vi "rsscope_core_global.vi"() -> ()   [LabVIEW 2018] (continued)
condition In Range or Out of Range.\n\nAvailable Repeated Capabilities:\nTrigger: TrigA, TrigB, TrigR\r\n\nRemote-control command(s):\nTRIGger<m>:DPHY:ESINdex:MAX"}, {"Level"=3, "Class Only"=TRUE, "Identifier"="", "Descriptive Name"="Escape Mode", "Data Type"=0, "Command"="", "Access"=0, "Range Table"="", "Read Callback"="", "Write Callback"="", "Supported Models"="", "Instrument Options"="", "Flags"=0, "Help"="Set the specified data value to be triggered on.The escape mode setup consists of the condition and one or two data patterns."}, {"Level"=4, "Class Only"=FALSE, "Identifier"="RSSCOPE_ATTR_DPHY_TRIGGER_ESCAPE_MODE_CONDITION", "Descriptive Name"="DPHY Trigger Escape Mode Condition", "Data Type"=0, "Command"="TRIG{Trigger}:DPHY:ESCM:COND", "Access"=2, "Range Table"="rsscope_rngProtocolTriggerCondition", "Read Callback"="", "Write Callback"="", "Supported Models"="", "Instrument Options"="K42", "Flags"=0, "Help"="Set the condition for the escape mode. You can define an exact value or a value range.\n\nAvailable Repeated Capabilities:\nTrigger: TrigA, TrigB, TrigR\r\n\nRemote-control command(s):\nTRIGger<m>:DPHY:ESCMode:CONDition"}, {"Level"=4, "Class Only"=FALSE, "Identifier"="RSSCOPE_ATTR_DPHY_TRIGGER_ESCAPE_MODE_MIN", "Descriptive Name"="DPHY Trigger Escape Mode Min", "Data Type"=2, "Command"="TRIG{Trigger}:DPHY:ESCM:MIN", "Access"=2, "Range Table"="", "Read Callback"="", "Write Callback"="", "Supported Models"="", "Instrument Options"="K42", "Flags"=0, "Help"="Specifies a escape mode bit pattern, or sets the start value of a pattern range.\n\nValid Values:\nBinary pattern string consisting of 1; 0; or X (any bit).\n\nAvailable Repeated Capabilities:\nTrigger: TrigA, TrigB, TrigR\r\n\nRemote-control command(s):\nTRIGger<m>:DPHY:ESCMode:MIN"}, {"Level"=4, "Class Only"=FALSE, "Identifier"="RSSCOPE_ATTR_DPHY_TRIGGER_ESCAPE_MODE_MAX", "Descriptive Name"="DPHY Trigger Escape Mode Max", "Data Type"=2, "Command"="TRIG{Trigger}:DPHY:ESCM:MAX", "Access"=2, "Range Table"="", "Read Callback"="", "Write Callback"="", "Supported Models"="", "Instrument Options"="K42", "Flags"=0, "Help"="Sets the end value of an escape mode range for condition In Range or Out of Range. \n\nValid Values:\nBinary pattern string consisting of 1; 0; or X (any bit).\n\nAvailable Repeated Capabilities:\nTrigger: TrigA, TrigB, TrigR\r\n\nRemote-control command(s):\nTRIGger<m>:DPHY:ESCMode:MAX"}, {"Level"=2, "Class Only"=TRUE, "Identifier"="", "Descriptive Name"="M-PHY", "Data Type"=0, "Command"="", "Access"=0, "Range Table"="", "Read Callback"="", "Write Callback"="", "Supported Models"="", "Instrument Options"="", "Flags"=0, "Help"="Contains attributes for M-PHY triggering."}, {"Level"=3, "Class Only"=FALSE, "Identifier"="RSSCOPE_ATTR_MPHY_TRIGGER_TYPE", "Descriptive Name"="MPHY Trigger Type", "Data Type"=0, "Command"="TRIG{Trigger}:MPHY:TYPE", "Access"=2, "Range Table"="RsScope_rngTriggerMPHYType", "Read Callback"="", "Write Callback"="", "Supported Models"="", "Instrument Options"="K44", "Flags"=0, "Help"="Selects the type of frame to be triggered on.\n\nAvailable Repeated Capabilities:\nTrigger: TrigA, TrigB, TrigR\r\n\nRemote-control command(s):\nTRIGger<m>:MPHY:TYPE"}, {"Level"=3, "Class Only"=FALSE, "Identifier"="RSSCOPE_ATTR_MPHY_TRIGGER_LCC_TYPE", "Descriptive Name"="MPHY Trigger LCC Type", "Data Type"=0, "Command"="TRIG{Trigger}:MPHY:LCCT", "Access"=2, "Range Table"="RsScope_rngTrigerMPHYLCCType", "Read Callback"="", "Write Callback"="", "Supported Models"="", "Instrument Options"="K44", "Flags"=0, "Help"="Selects the type of LCC frame to be triggered on.\n\nAvailable Repeated Capabilities:\nTrigger: TrigA, TrigB, TrigR\r\n\nRemote-control command(s):\nTRIGger<m>:MPHY:LCCType"}, {"Level"=3, "Class Only"=FALSE, "Identifier"="RSSCOPE_ATTR_MPHY_TRIGGER_WORD_ONE_CONDITION", "Descriptive Name"="MPHY Trigger Word One Condition", "Data Type"=0, "Command"="TRIG{Trigger}:MPHY:LWON:COND", "Access"=2, "Range Table"="rsscope_rngProtocolTriggerCondition", "Read Callback"="", "Write Callback"="", "Supported Models"="", "Instrument Options"="K44", "Flags"=0, "Help"="Sets the condition for WORD 1. You can define an exact value or a value range.\n\nAvailable Repeated Capabilities:\nTrigger: TrigA, TrigB, TrigR\r\n\nRemote-control command(s):\nTRIGger<m>:MPHY:LWONe:CONDition"}, {"Level"=3, "Class Only"=FALSE, "Identifier"="RSSCOPE_ATTR_MPHY_TRIGGER_WORD_ONE_MIN", "Descriptive Name"="MPHY Trigger Word One Min", "Data Type"=2, "Command"="TRIG{Trigger}:MPHY:LWON:MIN", "Access"=2, "Range Table"="", "Read Callback"="", "Write Callback"="", "Supported Models"="", "Instrument Options"="K44", "Flags"=0, "Help"="Specifies the WORD 1 pattern, or sets the start value of a pattern range.\n\nAvailable Repeated Capabilities:\nTrigger: TrigA, TrigB, TrigR\r\n\nRemote-control command(s):\nTRIGger<m>:MPHY:LWONe:MIN"}, {"Level"=3, "Class Only"=FALSE, "Identifier"="RSSCOPE_ATTR_MPHY_TRIGGER_WORD_ONE_MAX", "Descriptive Name"="MPHY Trigger Word One Max", "Data Type"=2, "Command"="TRIG{Trigger}:MPHY:LWON:MAX", "Access"=2, "Range Table"="", "Read Callback"="", "Write Callback"="", "Supported Models"="", "Instrument Options"="K44", "Flags"=0, "Help"="Sets the end value of the WORD 1 range if TRIGger<m>:MPHY:LWONe:CONDition is set to In Range or Out Of Range.\n\nAvailable Repeated Capabilities:\nTrigger: TrigA, TrigB, TrigR\r\n\nRemote-control command(s):\nTRIGger<m>:MPHY:LWONe:MAX"}, {"Level"=3, "Class Only"=FALSE, "Identifier"="RSSCOPE_ATTR_MPHY_TRIGGER_WORD_TWO_CONDITION", "Descriptive Name"="MPHY Trigger Word Two Condition", "Data Type"=0, "Command"="TRIG{Trigger}:MPHY:LWTW:COND", "Access"=2, "Range Table"="rsscope_rngProtocolTriggerCondition", "Read Callback"="", "Write Callback"="", "Supported Models"="", "Instrument Options"="K44", "Flags"=0, "Help"="Sets the condition for WORD 2. You can define an exact value or a value range.\n\nAvailable Repeated Capabilities:\nTrigger: TrigA, TrigB, TrigR\r\n\nRemote-control command(s):\nTRIGger<m>:MPHY:LWTWo:CONDition"}, {"Level"=3, "Class Only"=FALSE, "Identifier"="RSSCOPE_ATTR_MPHY_TRIGGER_WORD_TWO_MIN", "Descriptive Name"="MPHY Trigger Word Two Min", "Data Type"=2, "Command"="TRIG{Trigger}:MPHY:LWTW:MIN", "Access"=2, "Range Table"="", "Read Callback"="", "Write Callback"="", "Supported Models"="", "Instrument Options"="K44", "Flags"=0, "Help"="Specifies the WORD 2 pattern, or sets the start value of a pattern range.\n\nAvailable Repeated Capabilities:\nTrigger: TrigA, TrigB, TrigR\r\n\nRemote-control command(s):\nTRIGger<m>:MPHY:LWTWo:MIN"}, {"Level"=3, "Class Only"=FALSE, "Identifier"="RSSCOPE_ATTR_MPHY_TRIGGER_WORD_TWO_MAX", "Descriptive Name"="MPHY Trigger Word Two Max", "Data Type"=2, "Command"="TRIG{Trigger}:MPHY:LWTW:MAX", "Access"=2, "Range Table"="", "Read Callback"="", "Write Callback"="", "Supported Models"="", "Instrument Options"="K44", "Flags"=0, "Help"="Sets the end value of the WORD 2 range if TRIGger<m>:MPHY:LWTWo:CONDition is set to In Range or Out Of Range.\n\nAvailable Repeated Capabilities:\nTrigger: TrigA, TrigB, TrigR\r\n\nRemote-control command(s):\nTRIGger<m>:MPHY:LWTWo:MAX"}, {"Level"=3, "Class Only"=FALSE, "Identifier"="RSSCOPE_ATTR_MPHY_TRIGGER_WORD_THREE_CONDITION", "Descriptive Name"="MPHY Trigger Word Three Condition", "Data Type"=0, "Command"="TRIG{Trigger}:MPHY:LWTH:COND", "Access"=2, "Range Table"="rsscope_rngProtocolTriggerCondition", "Read Callback"="", "Write Callback"="", "Supported Models"="", "Instrument Options"="K44", "Flags"=0, "Help"="Sets the condition for WORD 3. You can define an exact value or a value range.\n\nAvailable Repeated Capabilities:\nTrigger: TrigA, TrigB, TrigR\r\n\nRemote-control command(s):\nTRIGger<m>:MPHY:LWTHree:CONDition"}, {"Level"=3, "Class Only"=FALSE, "Identifier"="RSSCOPE_ATTR_MPHY_TRIGGER_WORD_THREE_MIN", "Descriptive Name"="MPHY Trigger Word Three Min", "Data Type"=2, "Command"="TRIG{Trigger}:MPHY:LWTH:MIN", "Access"=2, "Range Table"="", "Read Callback"="", "Write Callback"="", "Supported Models"="", "Instrument Options"="K44", "Flags"=0, "Help"="Specifies the WORD 3 pattern, or sets the start value of a pattern range.\n\nAvailable Repeated Capabilities:\nTrigger: TrigA, TrigB, TrigR\r\n\nRemote-control command(s):\nTRIGger<m>:MPHY:LWTHree:MIN"}, {"Level"=3, "Class Only"=FALSE, "Identifier"="RSSCOPE_ATTR_MPHY_TRIGGER_WORD_THREE_MAX", "Descriptive Name"="MPHY Trigger Word Three Max", "Data Type"=2, "Command"="TRIG{Trigger}:MPHY:LWTH:MAX", "Access"=2, "Range Table"="", "Read Callback"="", "Write Callback"="", "Supported Models"="", "Instrument Options"="K44", "Flags"=0, "Help"="Sets the end value of the WORD 3 range if TRIGger<m>:MPHY:LWTHree:CONDition is set to In Range or Out Of Range.\n\nAvailable Repeated Capabilities:\nTrigger: TrigA, TrigB, TrigR\r\n\nRemote-control command(s):\nTRIGger<m>:MPHY:LWTHree:MAX"}, {"Level"=3, "Class Only"=FALSE, "Identifier"="RSSCOPE_ATTR_MPHY_TRIGGER_WORD_FOUR_CONDITION", "Descriptive Name"="MPHY Trigger Word Four Condition", "Data Type"=0, "Command"="TRIG{Trigger}:MPHY:LWF:COND", "Access"=2, "Range Table"="rsscope_rngProtocolTriggerCondition", "Read Callback"="", "Write Callback"="", "Supported Models"="", "Instrument Options"="K44", "Flags"=0, "Help"="Sets the condition for WORD 4. You can define an exact value or a value range.\n\nAvailable Repeated Capabilities:\nTrigger: TrigA, TrigB, TrigR\r\n\nRemote-control command(s):\nTRIGger<m>:MPHY:LWFour:CONDition"}, {"Level"=3, "Class Only"=FALSE, "Identifier"="RSSCOPE_ATTR_MPHY_TRIGGER_WORD_FOUR_MIN", "Descriptive Name"="MPHY Trigger Word Four Min", "Data Type"=2, "Command"="TRIG{Trigger}:MPHY:LWF:MIN", "Access"=2, "Range Table"="", "Read Callback"="", "Write Callback"="", "Supported Models"="", "Instrument Options"="K44", "Flags"=0, "Help"="Specifies the WORD 3 pattern, or sets the start value of a pattern range.\n\nAvailable Repeated Capabilities:\nTrigger: TrigA, TrigB, TrigR\r\n\nRemote-control command(s):\nTRIGger<m>:MPHY:LWFour:MIN"}, {"Level"=3, "Class Only"=FALSE, "Identifier"="RSSCOPE_ATTR_MPHY_TRIGGER_WORD_FOUR_MAX", "Descriptive Name"="MPHY Trigger Word Four Max", "Data Type"=2, "Command"="TRIG{Trigger}:MPHY:LWF:MAX", "Access"=2, "Range Table"="", "Read Callback"="", "Write Callback"="", "Supported Models"="", "Instrument Options"="K44", "Flags"=0, "Help"="Sets the end value of the WORD 4 range if TRIGger<m>:MPHY:LWFour:CONDition is set to In Range or Out Of Range.\n\nAvailable Repeated Capabilities:\nTrigger: TrigA, TrigB, TrigR\r\n\nRemote-control command(s):\nTRIGger<m>:MPHY:LWFour:MAX"}, {"Level"=3, "Class Only"=FALSE, "Identifier"="RSSCOPE_ATTR_MPHY_TRIGGER_TC_PATTERN", "Descriptive Name"="MPHY Trigger TC Pattern", "Data Type"=2, "Command"="TRIG{Trigger}:MPHY:TC", "Access"=2, "Range Table"="", "Read Callback"="", "Write Callback"="", "Supported Models"="", "Instrument Options"="K44", "Flags"=0, "Help"="Specifies the TC bit pattern.\n\nAvailable Repeated Capabilities:\nTrigger: TrigA, TrigB, TrigR\r\n\nRemote-control command(s):\nTRIGger<m>:MPHY:TC"}, {"Level"=3, "Class Only"=FALSE, "Identifier"="RSSCOPE_ATTR_MPHY_TRIGGER_DATA_CONDITION", "Descriptive Name"="MPHY Trigger Data Condition", "Data Type"=0, "Command"="TRIG{Trigger}:MPHY:DATA:DCON", "Access"=2, "Range Table"="rsscope_rngProtocolTriggerCondition", "Read Callback"="", "Write Callback"="", "Supported Models"="", "Instrument Options"="K44", "Flags"=0, "Help"="Sets the condition for the data. You can define an exact value or a value range.\n\nAvailable Repeated Capabilities:\nTrigger: TrigA, TrigB, TrigR\r\n\nRemote-control command(s):\nTRIGger<m>:MPHY:DATA:DCON"}, {"Level"=3, "Class Only"=FALSE, "Identifier"="RSSCOPE_ATTR_MPHY_TRIGGER_DATA_MIN", "Descriptive Name"="MPHY Trigger Data Min", "Data Type"=2, "Command"="TRIG{Trigger}:MPHY:DATA:DMIN", "Access"=2, "Range Table"="", "Read Callback"="", "Write Callback"="", "Supported Models"="", "Instrument Options"="K44", "Flags"=0, "Help"="Specifies the data bit pattern, or sets the start value of a pattern range.\n\nAvailable Repeated Capabilities:\nTrigger: TrigA, TrigB, TrigR\r\n\nRemote-control command(s):\nTRIGger<m>:MPHY:DATA:DMIN"}, {"Level"=3, "Class Only"=FALSE, "Identifier"="RSSCOPE_ATTR_MPHY_TRIGGER_DATA_MAX", "Descriptive Name"="MPHY Trigger Data Max", "Data Type"=2, "Command"="TRIG{Trigger}:MPHY:DATA:DMAX", "Access"=2, "Range Table"="", "Read Callback"="", "Write Callback"="", "Supported Models"="", "Instrument Options"="K44", "Flags"=0, "Help"="Sets the end value of the data range if TRIGger<m>:MPHY:DATA:DCON is set to In Range or Out Of Range.\n\nAvailable Repeated Capabilities:\nTrigger: TrigA, TrigB, TrigR\r\n\nRemote-control command(s):\nTRIGger<m>:MPHY:DATA:DMAX"}, {"Level"=3, "Class Only"=FALSE, "Identifier"="RSSCOPE_ATTR_MPHY_TRIGGER_INDEX_CONDITION", "Descriptive Name"="MPHY Trigger Index Condition", "Data Type"=0, "Command"="TRIG{Trigger}:MPHY:DATA:ICON", "Access"=2, "Range Table"="rsscope_rngProtocolTriggerCondition", "Read Callback"="", "Write Callback"="", "Supported Models"="", "Instrument Options"="K44", "Flags"=0, "Help"="Sets the condition for the index. You can define an exact value or a value range.\n\nAvailable Repeated Capabilities:\nTrigger: TrigA, TrigB, TrigR\r\n\nRemote-control command(s):\nTRIGger<m>:MPHY:DATA:ICONdition"}, {"Level"=3, "Class Only"=FALSE, "Identifier"="RSSCOPE_ATTR_MPHY_TRIGGER_INDEX_MIN", "Descriptive Name"="MPHY Trigger Index Min", "Data Type"=0, "Command"="TRIG{Trigger}:MPHY:DATA:IMIN", "Access"=2, "Range Table"="RsScope_rngMPHYTriggerIndex", "Read Callback"="", "Write Callback"="", "Supported Models"="", "Instrument Options"="K44", "Flags"=0, "Help"="Specifies the index minimum, or sets the start value of a range.\n\nAvailable Repeated Capabilities:\nTrigger: TrigA, TrigB, TrigR\r\n\nRemote-control command(s):\nTRIGger<m>:MPHY:DATA:IMIN"}, {"Level"=3, "Class Only"=FALSE, "Identifier"="RSSCOPE_ATTR_MPHY_TRIGGER_INDEX_MAX", "Descriptive Name"="MPHY Trigger Index Max", "Data Type"=0, "Command"="TRIG{Trigger}:MPHY:DATA:IMAX", "Access"=2, "Range Table"="RsScope_rngMPHYTriggerIndex", "Read Callback"="", "Write Callback"="", "Supported Models"="", "Instrument Options"="K44", "Flags"=0, "Help"="Sets the end value of the index range if TRIGger<m>:MPHY:DATA:ICON is set to INRange or RANge.\n\nAvailable Repeated Capabilities:\nTrigger: TrigA, TrigB, TrigR\r\n\nRemote-control command(s):\nTRIGger<m>:MPHY:DATA:IMAX"}, {"Level"=3, "Class Only"=FALSE, "Identifier"="RSSCOPE_ATTR_MPHY_TRIGGER_FSN_CONDITION", "Descriptive Name"="MPHY Trigger FSN Condition", "Data Type"=0, "Command"="TRIG{Trigger}:MPHY:FSN:COND", "Access"=2, "Range Table"="rsscope_rngProtocolTriggerCondition", "Read Callback"="", "Write Callback"="", "Supported Models"="", "Instrument Options"="K44", "Flags"=0, "Help"="Sets the condition for FSN. You can define an exact value or a value range.\n\nAvailable Repeated Capabilities:\nTrigger: TrigA, TrigB, TrigR\r\n\nRemote-control command(s):\nTRIGger<m>:MPHY:FSNumber:CONDition"}, {"Level"=3, "Class Only"=FALSE, "Identifier"="RSSCOPE_ATTR_MPHY_TRIGGER_FSN_MIN", "Descriptive Name"="MPHY Trigger FSN Min", "Data Type"=2, "Command"="TRIG{Trigger}:MPHY:FSN:MIN", "Access"=2, "Range Table"="", "Read Callback"="", "Write Callback"="", "Supported Models"="", "Instrument Options"="K44", "Flags"=0, "Help"="Specifies the FSN bit pattern, or sets the start value of a pattern range.\n\nAvailable Repeated Capabilities:\nTrigger: TrigA, TrigB, TrigR\r\n\nRemote-control command(s):\nTRIGger<m>:MPHY:FSNumber:MIN"}, {"Level"=3, "Class Only"=FALSE, "Identifier"="RSSCOPE_ATTR_MPHY_TRIGGER_FSN_MAX", "Descriptive Name"="MPHY Trigger FSN Max", "Data Type"=2, "Command"="TRIG{Trigger}:MPHY:FSN:MAX", "Access"=2, "Range Table"="", "Read Callback"="", "Write Callback"="", "Supported Models"="", "Instrument Options"="K44", "Flags"=0, "Help"="Sets the end value of the FSN range if TRIGger<m>:MPHY:FSNumber:CONDition is set to In Range or Out Of Range.\n\nAvailable Repeated Capabilities:\nTrigger: TrigA, TrigB, TrigR\r\n\nRemote-control command(s):\nTRIGger<m>:MPHY:FSNumber:MAX"}, {"Level"=3, "Class Only"=FALSE, "Identifier"="RSSCOPE_ATTR_MPHY_TRIGGER_CRC_CONDITION", "Descriptive Name"="MPHY Trigger CRC Condition", "Data Type"=0, "Command"="TRIG{Trigger}:MPHY:CRC:COND", "Access"=2, "Range Table"="rsscope_rngProtocolTriggerCondition", "Read Callback"="", "Write Callback"="", "Supported Models"="", "Instrument Options"="K44", "Flags"=0, "Help"="Sets the condition for CRC. You can define an exact value or a value range.\n\nAvailable Repeated Capabilities:\nTrigger: TrigA, TrigB, TrigR\r\n\nRemote-control command(s):\nTRIGger<m>:MPHY:CRC:CONDition"}, {"Level"=3, "Class Only"=FALSE, "Identifier"="RSSCOPE_ATTR_MPHY_TRIGGER_CRC_MIN", "Descriptive Name"="MPHY Trigger CRC Min", "Data Type"=2, "Command"="TRIG{Trigger}:MPHY:CRC:MIN", "Access"=2, "Range Table"="", "Read Callback"="", "Write Callback"="", "Supported Models"="", "Instrument Options"="K44", "Flags"=0, "Help"="Specifies the CRC bit pattern, or sets the start value of a pattern range.\n\nAvailable Repeated Capabilities:\nTrigger: TrigA, TrigB, TrigR\r\n\nRemote-control command(s):\nTRIGger<m>:MPHY:CRC:MIN"}, {"Level"=3, "Class Only"=FALSE, "Identifier"="RSSCOPE_ATTR_MPHY_TRIGGER_CRC_MAX", "Descriptive Name"="MPHY Trigger CRC Max", "Data Type"=2, "Command"="TRIG{Trigger}:MPHY:CRC:MAX", "Access"=2, "Range Table"="", "Read Callback"="", "Write Callback"="", "Supported Models"="", "Instrument Options"="K44", "Flags"=0, "Help"="Sets the end value of the CRC range if TRIGger<m>:MPHY:CRC:CONDition is set to In Range or Out Of Range.\n\nAvailable Repeated Capabilities:\nTrigger: TrigA, TrigB, TrigR\r\n\nRemote-control command(s):\nTRIGger<m>:MPHY:CRC:MAX"}, {"Level"=3, "Class Only"=FALSE, "Identifier"="RSSCOPE_ATTR_MPHY_TRIGGER_CREQ_PATTERN", "Descriptive Name"="MPHY Trigger CREQ Pattern", "Data Type"=0, "Command"="TRIG{Trigger}:MPHY:CREQ", "Access"=2, "Range Table"="RsScope_rngMPHYREQPattern", "Read Callback"="", "Write Callback"="", "Supported Models"="", "Instrument Options"="K44", "Flags"=0, "Help"="Specifies the CREQ bit pattern.\n\nAvailable Repeated Capabilities:\nTrigger: TrigA, TrigB, TrigR\r\n\nRemote-control command(s):\nTRIGger<m>:MPHY:CREQ"}, {"Level"=3, "Class Only"=FALSE, "Identifier"="RSSCOPE_ATTR_MPHY_TRIGGER_RREQ_PATTERN", "Descriptive Name"="MPHY Trigger RREQ Pattern", "Data Type"=0, "Command"="TRIG{Trigger}:MPHY:RREQ", "Access"=2, "Range Table"="RsScope_rngMPHYREQPattern", "Read Callback"="", "Write Callback"="", "Supported Models"="", "Instrument Options"="K44", "Flags"=0, "Help"="Specifies the RREQ bit pattern.\n\nAvailable Repeated Capabilities:\nTrigger: TrigA, TrigB, TrigR\r\n\nRemote-control command(s):\nTRIGger<m>:MPHY:RREQ"}, {"Level"=3, "Class Only"=FALSE, "Identifier"="RSSCOPE_ATTR_MPHY_TRIGGER_CREDIT_CONDITION", "Descriptive Name"="MPHY Trigger Credit Condition", "Data Type"=0, "Command"="TRIG{Trigger}:MPHY:CRED:COND", "Access"=2, "Range Table"="rsscope_rngProtocolTriggerCondition", "Read Callback"="", "Write Callback"="", "Supported Models"="", "Instrument Options"="K44", "Flags"=0, "Help"="Sets the condition for Credit. You can define an exact value or a value range.\n\nAvailable Repeated Capabilities:\nTrigger: TrigA, TrigB, TrigR\r\n\nRemote-control command(s):\nTRIGger<m>:MPHY:CREDit:CONDition"}, {"Level"=3, "Class Only"=FALSE, "Identifier"="RSSCOPE_ATTR_MPHY_TRIGGER_CREDIT_MIN", "Descriptive Name"="MPHY Trigger Credit Min", "Data Type"=2, "Command"="TRIG{Trigger}:MPHY:CRED:MIN", "Access"=2, "Range Table"="", "Read Callback"="", "Write Callback"="", "Supported Models"="", "Instrument Options"="K44", "Flags"=0, "Help"="Specifies the Credit bit pattern, or sets the start value of a pattern range.\n\nAvailable Repeated Capabilities:\nTrigger: TrigA, TrigB, TrigR\r\n\nRemote-control command(s):\nTRIGger<m>:MPHY:CREDit:MIN"}, {"Level"=3, "Class Only"=FALSE, "Identifier"="RSSCOPE_ATTR_MPHY_TRIGGER_CREDIT_MAX", "Descriptive Name"="MPHY Trigger Credit Max", "Data Type"=2, "Command"="TRIG{Trigger}:MPHY:CRED:MAX", "Access"=2, "Range Table"="", "Read Callback"="", "Write Callback"="", "Supported Models"="", "Instrument Options"="K44", "Flags"=0, "Help"="Sets the end value of the Credit range if TRIGger<m>:MPHY:CREDit:CONDition is set to In Range or Out Of Range.\n\nAvailable Repeated Capabilities:\nTrigger: TrigA, TrigB, TrigR\r\n\nRemote-control command(s):\nTRIGger<m>:MPHY:CREDit:MAX"}, {"Level"=3, "Class Only"=FALSE, "Identifier"="RSSCOPE_ATTR_MPHY_TRIGGER_PACP_BEGIN_CONDITION", "Descriptive Name"="MPHY Trigger PACP Begin Condition", "Data Type"=0, "Command"="TRIG{Trigger}:MPHY:PBEG:COND", "Access"=2, "Range Table"="rsscope_rngProtocolTriggerCondition", "Read Callback"="", "Write Callback"="", "Supported Models"="", "Instrument Options"="K44", "Flags"=0, "Help"="Sets the condition for PACP Begin. You can define an exact value or a value range.\n\nAvailable Repeated Capabilities:\nTrigger: TrigA, TrigB, TrigR\r\n\nRemote-control command(s):\nTRIGger<m>:MPHY:PBEGin:CONDition"}, {"Level"=3, "Class Only"=FALSE, "Identifier"="RSSCOPE_ATTR_MPHY_TRIGGER_PACP_BEGIN_MIN", "Descriptive Name"="MPHY Trigger PACP Begin Min", "Data Type"=2, "Command"="TRIG{Trigger}:MPHY:PBEG:MIN", "Access"=2, "Range Table"="", "Read Callback"="", "Write Callback"="", "Supported Models"="", "Instrument Options"="K44", "Flags"=0, "Help"="Specifies the PACP Begin bit pattern, or sets the start value of a pattern range.\n\nAvailable Repeated Capabilities:\nTrigger: TrigA, TrigB, TrigR\r\n\nRemote-control command(s):\nTRIGger<m>:MPHY:PBEGin:MIN"}, {"Level"=3, "Class Only"=FALSE, "Identifier"="RSSCOPE_ATTR_MPHY_TRIGGER_PACP_BEGIN_MAX", "Descriptive Name"="MPHY Trigger PACP Begin Max", "Data Type"=2, "Command"="TRIG{Trigger}:MPHY:PBEG:MAX", "Access"=2, "Range Table"="", "Read Callback"="", "Write Callback"="", "Supported Models"="", "Instrument Options"="K44", "Flags"=0, "Help"="Sets the end value of the PACP Begin range if TRIGger<m>:MPHY:PBEGin:CONDition is set to In Range or Out Of Range.\n\nAvailable Repeated Capabilities:\nTrigger: TrigA, TrigB, TrigR\r\n\nRemote-control command(s):\nTRIGger<m>:MPHY:PBEGin:MAX"}, {"Level"=3, "Class Only"=FALSE, "Identifier"="RSSCOPE_ATTR_MPHY_TRIGGER_PACP_ID_CONDITION", "Descriptive Name"="MPHY Trigger PACP ID Condition", "Data Type"=0, "Command"="TRIG{Trigger}:MPHY:PFID:COND", "Access"=2, "Range Table"="rsscope_rngProtocolTriggerCondition", "Read Callback"="", "Write Callback"="", "Supported Models"="", "Instrument Options"="K44", "Flags"=0, "Help"="Sets the condition for PACP Function ID. You can define an exact value or a value range.\n\nAvailable Repeated Capabilities:\nTrigger: TrigA, TrigB, TrigR\r\n\nRemote-control command(s):\nTRIGger<m>:MPHY:PFID:CONDition"}, {"Level"=3, "Class Only"=FALSE, "Identifier"="RSSCOPE_ATTR_MPHY_TRIGGER_PACP_ID_MIN", "Descriptive Name"="MPHY Trigger PACP ID Min", "Data Type"=2, "Command"="TRIG{Trigger}:MPHY:PFID:MIN", "Access"=2, "Range Table"="", "Read Callback"="", "Write Callback"="", "Supported Models"="", "Instrument Options"="K44", "Flags"=0, "Help"="Specifies the PACP Function ID bit pattern, or sets the start value of a pattern range.\n\nAvailable Repeated Capabilities:\nTrigger: TrigA, TrigB, TrigR\r\n\nRemote-control command(s):\nTRIGger<m>:MPHY:PFID:MIN"}, {"Level"=3, "Class Only"=FALSE, "Identifier"="RSSCOPE_ATTR_MPHY_TRIGGER_PACP_ID_MAX", "Descriptive Name"="MPHY Trigger PACP ID Max", "Data Type"=2, "Command"="TRIG{Trigger}:MPHY:PFID:MAX", "Access"=2, "Range Table"="", "Read Callback"="", "Write Callback"="", "Supported Models"="", "Instrument Options"="K44", "Flags"=0, "Help"="Sets the end value of the PACP Function ID range if TRIGger<m>:MPHY:PFID:CONDition is set to In Range or Out Of Range.\n\nAvailable Repeated Capabilities:\nTrigger: TrigA, TrigB, TrigR\r\n\nRemote-control command(s):\nTRIGger<m>:MPHY:PFID:MAX"}, {"Level"=3, "Class Only"=FALSE, "Identifier"="RSSCOPE_ATTR_MPHY_TRIGGER_PRP_WIDTH", "Descriptive Name"="MPHY Trigger PRP Width", "Data Type"=1, "Command"="TRIG{Trigger}:MPHY:PRPL", "Access"=2, "Range Table"="RsScope_rngMPHYTriggerPRPWidth", "Read Callback"="", "Write Callback"="", "Supported Models"="", "Instrument Options"="K44", "Flags"=0, "Help"="Sets the width for the width trigger based upon the data rate.\n\nAvailable Repeated Capabilities:\nTrigger: TrigA, TrigB, TrigR\r\n\nRemote-control command(s):\nTRIGger<m>:MPHY:PRPLength"}, {"Level"=3, "Class Only"=FALSE, "Identifier"="RSSCOPE_ATTR_MPHY_TRIGGER_LCC_ERROR", "Descriptive Name"="MPHY Trigger LCC Error", "Data Type"=3, "Command"="TRIG{Trigger}:MPHY:ERR:LCMD", "Access"=2, "Range Table"="", "Read Callback"="", "Write Callback"="", "Supported Models"="", "Instrument Options"="K44", "Flags"=0, "Help"="Enables or disables trigger on LCC error.\n\nAvailable Repeated Capabilities:\nTrigger: TrigA, TrigB, TrigR\r\n\nRemote-control command(s):\nTRIGger<m>:MPHY:ERRor:LCMD"}, {"Level"=3, "Class Only"=FALSE, "Identifier"="RSSCOPE_ATTR_MPHY_TRIGGER_ERROR_LENGTH", "Descriptive Name"="MPHY Trigger Error Length", "Data Type"=3, "Command"="TRIG{Trigger}:MPHY:ERR:LENG", "Access"=2, "Range Table"="", "Read Callback"="", "Write Callback"="", "Supported Models"="", "Instrument Options"="K44", "Flags"=0, "Help"="Enables or disables trigger on length error.\n\nAvailable Repeated Capabilities:\nTrigger: TrigA, TrigB, TrigR\r\n\nRemote-control command(s):\nTRIGger<m>:MPHY:ERRor:LENGth"}, {"Level"=3, "Class Only"=FALSE, "Identifier"="RSSCOPE_ATTR_MPHY_TRIGGER_ERROR_RESERVED", "Descriptive Name"="MPHY Trigger Error Reserved", "Data Type"=3, "Command"="TRIG{Trigger}:MPHY:ERR:RES", "Access"=2, "Range Table"="", "Read Callback"="", "Write Callback"="", "Supported Models"="", "Instrument Options"="K44", "Flags"=0, "Help"="Enables or disables trigger on reserved bit error.\n\nAvailable Repeated Capabilities:\nTrigger: TrigA, TrigB, TrigR\r\n\nRemote-control command(s):\nTRIGger<m>:MPHY:ERRor:REServed"}, {"Level"=3, "Class Only"=FALSE, "Identifier"="RSSCOPE_ATTR_MPHY_TRIGGER_ERROR_SYMBOL", "Descriptive Name"="MPHY Trigger Error Symbol", "Data Type"=3, "Command"="TRIG{Trigger}:MPHY:ERR:SYMB", "Access"=2, "Range Table"="", "Read Callback"="", "Write Callback"="", "Supported Models"="", "Instrument Options"="K44", "Flags"=0, "Help"="Enables or disables trigger on 8b10b symbol error.\n\nAvailable Repeated Capabilities:\nTrigger: TrigA, TrigB, TrigR\r\n\nRemote-control command(s):\nTRIGger<m>:MPHY:ERRor:SYMBol"}, {"Level"=3, "Class Only"=FALSE, "Identifier"="RSSCOPE_ATTR_MPHY_TRIGGER_ERROR_UNIDENTIFIED_UNIPRO_FRAME", "Descriptive Name"="MPHY Trigger Error Unidentified UniPro Frame", "Data Type"=3, "Command"="TRIG{Trigger}:MPHY:ERR:UNKN", "Access"=2, "Range Table"="", "Read Callback"="", "Write Callback"="", "Supported Models"="", "Instrument Options"="K44", "Flags"=0, "Help"="Enables or disables trigger on unidentified UniPro frame error.\n\nAvailable Repeated Capabilities:\nTrigger: TrigA, TrigB, TrigR\r\n\nRemote-control command(s):\nTRIGger<m>:MPHY:ERRor:UNKNown"}, {"Level"=3, "Class Only"=TRUE, "Identifier"="", "Descriptive Name"="SSIC", "Data Type"=0, "Command"="", "Access"=0, "Range Table"="", "Read Callback"="", "Write Callback"="", "Supported Models"="", "Instrument Options"="", "Flags"=0, "Help"="Trigger Settings MPHY SSIC"}, {"Level"=2, "Class Only"=TRUE, "Identifier"="", "Descriptive Name"="Space Wire", "Data Type"=0, "Command"="", "Access"=0, "Range Table"="", "Read Callback"="", "Write Callback"="", "Supported Models"="", "Instrument Options"="", "Flags"=0, "Help"="Configures Space Wire trigger."}, {"Level"=3, "Class Only"=FALSE, "Identifier"="RSSCOPE_ATTR_SPACE_WIRE_TRIGGER_TYPE", "Descriptive Name"="Space Wire Trigger Type", "Data Type"=0, "Command"="TRIG{Trigger}:SWIR:TYPE", "Access"=2, "Range Table"="RsScope_rngSpaceWireTriggerType", "Read Callback"="", "Write Callback"="", "Supported Models"="", "Instrument Options"="K65", "Flags"=0, "Help"="Sets the trigger type for the Space Wire analysis.\n\nAvailable Repeated Capabilities:\nTrigger: TrigA, TrigB, TrigR\r\n\nRemote-control command(s):\nTRIGger<m>:SWIRe:TYPE"}, {"Level"=3, "Class Only"=FALSE, "Identifier"="RSSCOPE_ATTR_SPACE_WIRE_TRIGGER_CONTROL_TYPE", "Descriptive Name"="Space Wire Trigger Control Type", "Data Type"=0, "Command"="TRIG{Trigger}:SWIR:CTYP", "Access"=2, "Range Table"="RsScope_rngSpaceWireTriggerControlType", "Read Callback"="", "Write Callback"="", "Supported Models"="", "Instrument Options"="K65", "Flags"=0, "Help"="Triggers on a specific control type character.\n\nAvailable Repeated Capabilities:\nTrigger: TrigA, TrigB, TrigR\r\n\nRemote-control command(s):\nTRIGger<m>:SWIRe:CTYPe"}, {"Level"=3, "Class Only"=TRUE, "Identifier"="", "Descriptive Name"="Time Code", "Data Type"=0, "Command"="", "Access"=0, "Range Table"="", "Read Callback"="", "Write Callback"="", "Supported Models"="", "Instrument Options"="", "Flags"=0, "Help"="Sets the specified data type for the time code to be triggered on. The data type setup consists of the condition and one or two data patterns."}, {"Level"=4, "Class Only"=FALSE, "Identifier"="RSSCOPE_ATTR_SPACE_WIRE_TRIGGER_TIME_CODE_CONDITION", "Descriptive Name"="Space Wire Trigger Time Code Condition", "Data Type"=0, "Command"="TRIG{Trigger}:SWIR:TIME:COND", "Access"=2, "Range Table"="rsscope_rngProtocolTriggerCondition", "Read Callback"="", "Write Callback"="", "Supported Models"="", "Instrument Options"="K65", "Flags"=0, "Help"="Set the condition for the data value for the time code. You can define an exact value or a value range.\n\nAvailable Repeated Capabilities:\nTrigger: TrigA, TrigB, TrigR\r\n\nRemote-control command(s):\nTRIGger<m>:SWIRe:TIME:CONDition"}, {"Level"=4, "Class Only"=FALSE, "Identifier"="RSSCOPE_ATTR_SPACE_WIRE_TRIGGER_TIME_CODE_MIN", "Descriptive Name"="Space Wire Trigger Time Code Min", "Data Type"=2, "Command"="TRIG{Trigger}:SWIR:TIME:MIN", "Access"=2, "Range Table"="", "Read Callback"="", "Write Callback"="", "Supported Models"="", "Instrument Options"="K65", "Flags"=0, "Help"="Specifies a pattern for the data value for the time code, or sets the start value of a pattern range.\n\nValid Values:\nBinary pattern string consisting of 1; 0; or X (any bit).\n\nAvailable Repeated Capabilities:\nTrigger: TrigA, TrigB, TrigR\r\n\nRemote-control command(s):\nTRIGger<m>:SWIRe:TIME:MIN"}, {"Level"=4, "Class Only"=FALSE, "Identifier"="RSSCOPE_ATTR_SPACE_WIRE_TRIGGER_TIME_CODE_MAX", "Descriptive Name"="Space Wire Trigger Time Code Max", "Data Type"=2, "Command"="TRIG{Trigger}:SWIR:TIME:MAX", "Access"=2, "Range Table"="", "Read Callback"="", "Write Callback"="", "Supported Models"="", "Instrument Options"="K65", "Flags"=0, "Help"="Sets the end value of a data value for the time code range for condition In Range or Out of Range. \n\nValid Values:\nBinary pattern string consisting of 1; 0; or X (any bit).\n\nAvailable Repeated Capabilities:\nTrigger: TrigA, TrigB, TrigR\r\n\nRemote-control command(s):\nTRIGger<m>:SWIRe:TIME:MAX"}, {"Level"=3, "Class Only"=TRUE, "Identifier"="", "Descriptive Name"="Data", "Data Type"=0, "Command"="", "Access"=0, "Range Table"="", "Read Callback"="", "Write Callback"="", "Supported Models"="", "Instrument Options"="", "Flags"=0, "Help"="Sets the specified data type for the data pattern to be triggered on. The data type setup consists of the condition and one or two data patterns."}, {"Level"=4, "Class Only"=FALSE, "Identifier"="RSSCOPE_ATTR_SPACE_WIRE_TRIGGER_DATA_CONDITION", "Descriptive Name"="Space Wire Trigger Data Condition", "Data Type"=0, "Command"="TRIG{Trigger}:SWIR:DATA:COND", "Access"=2, "Range Table"="rsscope_rngProtocolTriggerCondition", "Read Callback"="", "Write Callback"="", "Supported Models"="", "Instrument Options"="K65", "Flags"=0, "Help"="Set the condition for the data value. You can define an exact value or a value range.\n\nAvailable Repeated Capabilities:\nTrigger: TrigA, TrigB, TrigR\r\n\nRemote-control command(s):\nTRIGger<m>:SWIRe:DATA:CONDition"}, {"Level"=4, "Class Only"=FALSE, "Identifier"="RSSCOPE_ATTR_SPACE_WIRE_TRIGGER_DATA_MIN", "Descriptive Name"="Space Wire Trigger Data Min", "Data Type"=2, "Command"="TRIG{Trigger}:SWIR:DATA:MIN", "Access"=2, "Range Table"="", "Read Callback"="", "Write Callback"="", "Supported Models"="", "Instrument Options"="K65", "Flags"=0, "Help"="Specifies a data for the data pattern, or sets the start value of a pattern range.\n\nValid Values:\nBinary pattern string consisting of 1; 0; or X (any bit).\n\nAvailable Repeated Capabilities:\nTrigger: TrigA, TrigB, TrigR\r\n\nRemote-control command(s):\nTRIGger<m>:SWIRe:DATA:MIN"}, {"Level"=4, "Class Only"=FALSE, "Identifier"="RSSCOPE_ATTR_SPACE_WIRE_TRIGGER_DATA_MAX", "Descriptive Name"="Space Wire Trigger Data Max", "Data Type"=2, "Command"="TRIG{Trigger}:SWIR:DATA:MAX", "Access"=2, "Range Table"="", "Read Callback"="", "Write Callback"="", "Supported Models"="", "Instrument Options"="K65", "Flags"=0, "Help"="Sets the end value of a data for the data pattern range for condition In Range or Out of Range. \n\nValid Values:\nBinary pattern string consisting of 1; 0; or X (any bit).\n\nAvailable Repeated Capabilities:\nTrigger: TrigA, TrigB, TrigR\r\n\nRemote-control command(s):\nTRIGger<m>:SWIRe:DATA:MAX"}, {"Level"=3, "Class Only"=TRUE, "Identifier"="", "Descriptive Name"="Error", "Data Type"=0, "Command"="", "Access"=0, "Range Table"="", "Read Callback"="", "Write Callback"="", "Supported Models"="", "Instrument Options"="", "Flags"=0, "Help"="Triggers on a error."}, {"Level"=4, "Class Only"=FALSE, "Identifier"="RSSCOPE_ATTR_SPACE_WIRE_TRIGGER_PARITY_ERROR", "Descriptive Name"="Space Wire Trigger Parity Error", "Data Type"=3, "Command"="TRIG{Trigger}:SWIR:ERR:PAR", "Access"=2, "Range Table"="", "Read Callback"="", "Write Callback"="", "Supported Models"="", "Instrument Options"="K65", "Flags"=0, "Help"="Enables triggering on a parity error (even parity).\n\nAvailable Repeated Capabilities:\nTrigger: TrigA, TrigB, TrigR\r\n\nRemote-control command(s):\nTRIGger<m>:SWIRe:ERRor:PARity"}, {"Level"=4, "Class Only"=FALSE, "Identifier"="RSSCOPE_ATTR_SPACE_WIRE_TRIGGER_ESCAPE_ERROR", "Descriptive Name"="Space Wire Trigger Escape Error", "Data Type"=3, "Command"="TRIG{Trigger}:SWIR:ERR:ESC", "Access"=2, "Range Table"="", "Read Callback"="", "Write Callback"="", "Supported Models"="", "Instrument Options"="K65", "Flags"=0, "Help"="Enables trigger on an escape error.\n\nAvailable Repeated Capabilities:\nTrigger: TrigA, TrigB, TrigR\r\n\nRemote-control command(s):\nTRIGger<m>:SWIRe:ERRor:ESC"}, {"Level"=2, "Class Only"=TRUE, "Identifier"="", "Descriptive Name"="Zone", "Data Type"=0, "Command"="", "Access"=0, "Range Table"="", "Read Callback"="", "Write Callback"="", "Supported Models"="", "Instrument Options"="", "Flags"=0, "Help"="Contains attributes for Zone Triggering."}, {"Level"=3, "Class Only"=FALSE, "Identifier"="RSSCOPE_ATTR_ZONE_LOGICAL_EXPRESSION", "Descriptive Name"="Zone Logical Expression", "Data Type"=2, "Command"="TRIG:ZONE:EXPR", "Access"=2, "Range Table"="", "Read Callback"="", "Write Callback"="", "Supported Models"="", "Instrument Options"="K19", "Flags"=0, "Help"="Defines the zone trigger.\n\nAvailable Repeated Capabilities:\nNone\n\nRemote-control command(s):\nTRIGger<m>:ZONE:EXPRession[:DEFine]"}, {"Level"=3, "Class Only"=FALSE, "Identifier"="RSSCOPE_ATTR_APPLY_ZONE_TRIGGER_HISTORY", "Descriptive Name"="Apply Zone Trigger History", "Data Type"=3, "Command"="SWTR:HIST", "Access"=2, "Range Table"="", "Read Callback"="", "Write Callback"="", "Supported Models"="", "Instrument Options"="K19", "Flags"=0, "Help"="Applies the zone trigger condition to the acquisitions in the history memory during history replay.\n\nAvailable Repeated Capabilities:\nNone\n\nRemote-control command(s):\nSWTRigger:HISTory"}, {"Level"=2, "Class Only"=TRUE, "Identifier"="", "Descriptive Name"="CXPI", "Data Type"=0, "Command"="", "Access"=0, "Range Table"="", "Read Callback"="", "Write Callback"="", "Supported Models"="", "Instrument Options"="", "Flags"=0, "Help"="Configures CXPI trigger."}, {"Level"=3, "Class Only"=FALSE, "Identifier"="RSSCOPE_ATTR_CXPI_TRIGGER_TYPE", "Descriptive Name"="CXPI Trigger Type", "Data Type"=0, "Command"="TRIG{Trigger}:CXPI:TYPE", "Access"=2, "Range Table"="RsScope_rngCXPITriggerType", "Read Callback"="", "Write Callback"="", "Supported Models"="", "Instrument Options"="K76", "Flags"=0, "Help"="Selects the trigger type for the CXPI analysis.\n\nAvailable Repeated Capabilities:\nTrigger: TrigA, TrigB, TrigR\r\n\nRemote-control command(s):\nTRIGger<m>:CXPI:TYPE"}, {"Level"=3, "Class Only"=FALSE, "Identifier"="RSSCOPE_ATTR_CXPI_TRIGGER_NM", "Descriptive Name"="CXPI Trigger NM", "Data Type"=2, "Command"="TRIG{Trigger}:CXPI:NM", "Access"=2, "Range Table"="", "Read Callback"="", "Write Callback"="", "Supported Models"="", "Instrument Options"="K76", "Flags"=0, "Help"="Sets the value of the network management (NM) field.\n\nAvailable Repeated Capabilities:\nTrigger: TrigA, TrigB, TrigR\r\n\nRemote-control command(s):\nTRIGger<m>:CXPI:NM"}, {"Level"=3, "Class Only"=FALSE, "Identifier"="RSSCOPE_ATTR_CXPI_TRIGGER_CT", "Descriptive Name"="CXPI Trigger CT", "Data Type"=2, "Command"="TRIG{Trigger}:CXPI:CT", "Access"=2, "Range Table"="", "Read Callback"="", "Write Callback"="", "Supported Models"="", "Instrument Options"="K76", "Flags"=0, "Help"="Sets the value of the counter (CT), 2 bits indicating the continuity of the frame.\n\nAvailable Repeated Capabilities:\nTrigger: TrigA, TrigB, TrigR\r\n\nRemote-control command(s):\nTRIGger<m>:CXPI:CT"}, {"Level"=3, "Class Only"=TRUE, "Identifier"="", "Descriptive Name"="Frame ID", "Data Type"=0, "Command"="", "Access"=0, "Range Table"="", "Read Callback"="", "Write Callback"="", "Supported Models"="", "Instrument Options"="", "Flags"=0, "Help"="The frame identifier is a 7-bit field. Its setup consists of the condition and one or two frame patterns."}, {"Level"=4, "Class Only"=FALSE, "Identifier"="RSSCOPE_ATTR_CXPI_TRIGGER_FRAME_ID_CONDITION", "Descriptive Name"="CXPI Trigger Frame ID Condition", "Data Type"=0, "Command"="TRIG{Trigger}:CXPI:FID:COND", "Access"=2, "Range Table"="rsscope_rngProtocolTriggerCondition", "Read Callback"="", "Write Callback"="", "Supported Models"="", "Instrument Options"="K76", "Flags"=0, "Help"="Set the condition for the frame ID. You can define an exact value or a value range.\n\nAvailable Repeated Capabilities:\nTrigger: TrigA, TrigB, TrigR\r\n\nRemote-control command(s):\nTRIGger<m>:CXPI:FID:CONDition"}, {"Level"=4, "Class Only"=FALSE, "Identifier"="RSSCOPE_ATTR_CXPI_TRIGGER_FRAME_ID_MIN", "Descriptive Name"="CXPI Trigger Frame ID Min", "Data Type"=2, "Command"="TRIG{Trigger}:CXPI:FID:MIN", "Access"=2, "Range Table"="", "Read Callback"="", "Write Callback"="", "Supported Models"="", "Instrument Options"="K76", "Flags"=0, "Help"="Specifies a frame ID pattern, or sets the start value of a pattern range.\n\nValid Values:\nBinary pattern string consisting of 1; 0; or X (any bit).\n\nAvailable Repeated Capabilities:\nTrigger: TrigA, TrigB, TrigR\r\n\nRemote-control command(s):\nTRIGger<m>:CXPI:FID:MIN"}, {"Level"=4, "Class Only"=FALSE, "Identifier"="RSSCOPE_ATTR_CXPI_TRIGGER_FRAME_ID_MAX", "Descriptive Name"="CXPI Trigger Frame ID Max", "Data Type"=2, "Command"="TRIG{Trigger}:CXPI:FID:MAX", "Access"=2, "Range Table"="", "Read Callback"="", "Write Callback"="", "Supported Models"="", "Instrument Options"="K76", "Flags"=0, "Help"="Sets the end value of a frame ID range for condition In Range or Out of Range. \n\nValid Values:\nBinary pattern string consisting of 1; 0; or X (any bit).\n\nAvailable Repeated Capabilities:\nTrigger: TrigA, TrigB, TrigR\r\n\nRemote-control command(s):\nTRIGger<m>:CXPI:FID:MAX"}, {"Level"=3, "Class Only"=TRUE, "Identifier"="", "Descriptive Name"="DLC", "Data Type"=0, "Command"="", "Access"=0, "Range Table"="", "Read Callback"="", "Write Callback"="", "Supported Models"="", "Instrument Options"="", "Flags"=0, "Help"="Sets the data length code, which 
